vi "prepractica 6.vi"() -> ()   [LabVIEW 2015]
panel:
  in  "Entrada":dbl
  in  "Repeticiones":dbl
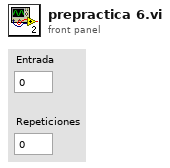
[diagram p1: front panel]
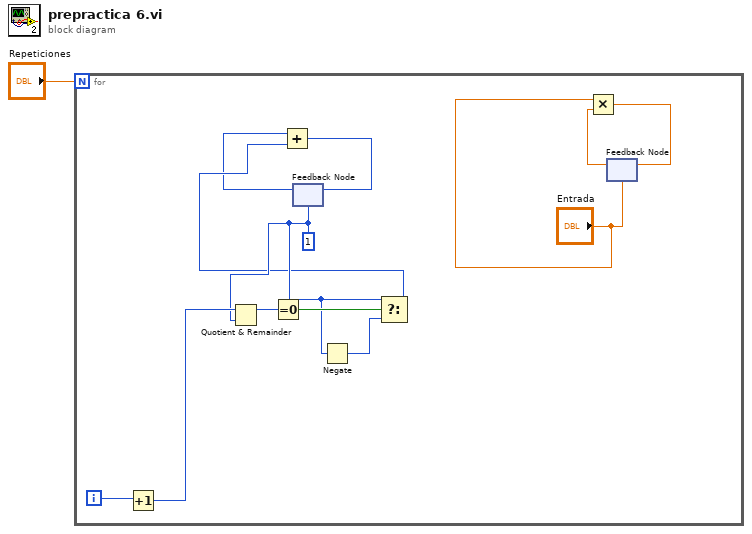
[diagram p0: block diagram]
diagram:
  n1 = for {
    N: "Repeticiones" -> [_]
    i -> [w13]
    w5 = 1
    n2 = Increment(x=w13) -> (x+1=w8:i32)
    n3 = Quotient & Remainder(x=w8, y=w5) -> (x-y*floor(x/y)=w7:i32)  [unwired: 1 out]
    n4 = Equal To 0?(x=w7) -> (x = 0?=w6:bool)
    n5 = feedback #1(w5) -> (w2:i32)
    n6 = Negate(x=w5) -> (-x=w4:i32)
    n7 = Select(t=w5, s=w6, f=w4) -> (s? t:f=w3:i32)
    n8 = Add(x=w2, y=w3) -> (x+y=w9:i32)
    n9 = feedback-in #1(w9) -> ()
    n10 = feedback #2("Entrada") -> (w12:dbl)
    n11 = Multiply(x="Entrada", y=w12) -> (x*y=w10:dbl)
    n12 = feedback-in #2(w10) -> ()
  }
